vi "CTRE_Phoenix_MotorControl_BufferedTrajectoryPointStream_Clear.vi"(8 "error in":errorcluster, 11 "BufferedTrajectoryPointStream_DevRef":T1) -> (0 "error out":errorcluster, 3 "BufferedTrajectoryPointStream_DevRef":T1)   [LabVIEW 2020]
doc: "Clears the Buffered Trajectory Point Stream"
uses:
  <vilib>/Rock Robotics/WPI/ThirdParty/Phoenix-LabVIEW/Motor Controller/Controls/CTRE_Phoenix_MotorControl_BufferedTrajectoryPointStream_DeviceRef.ctl
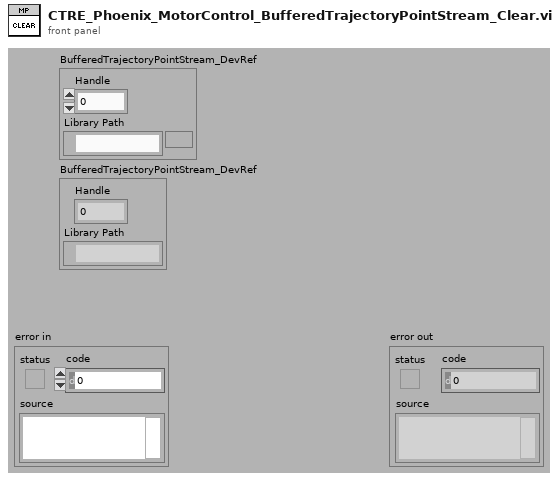
[diagram p1: front panel]
types:
  T1 = typedef "CTRE_Phoenix_MotorControl_BufferedTrajectoryPointStream_DeviceRef.ctl" = cluster{"Handle":u64, "Library Path":path}
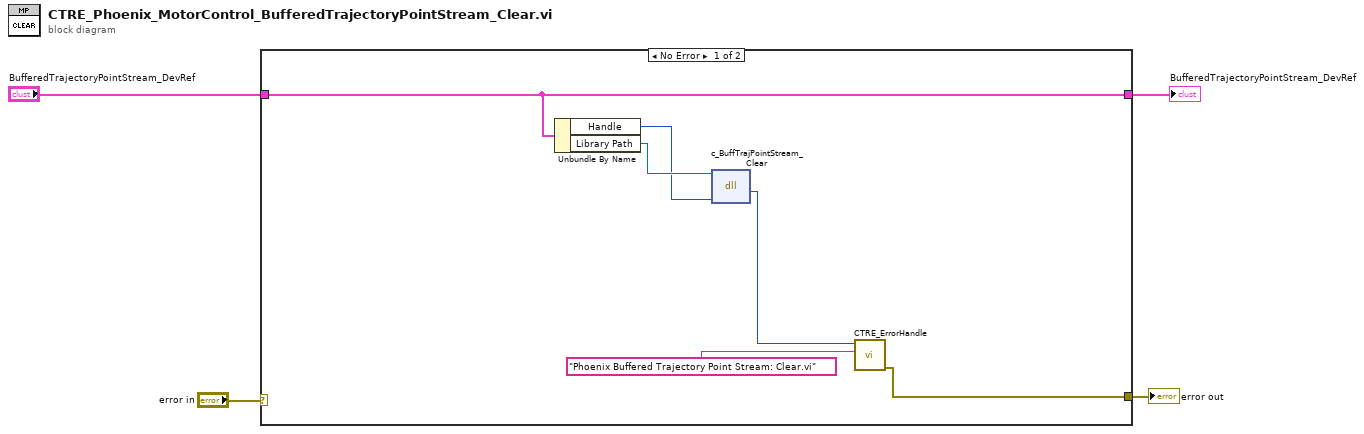
[diagram p0: block diagram]
diagram:
  n1 = case shown="No Error" "error in" {
    selector: "error in" -> [_ w12]
    tunnel: [w5 w12] -> w4
    tunnel: [w10 w11] -> w1
    tunnel: "BufferedTrajectoryPointStream_DevRef" -> [w10 w11]
    frame No Error {
      n2 = Unbundle By Name(w10) -> ("Handle"=w8:u64, "Library Path"=w9:path)
      n3 = dll-call lib="?" fn="c_BuffTrajPointStream_Clear"(path in=w9, "handle"=w8) -> ("ErrorCode"=w6:i32)  [unwired: 3 in, 2 out]
      n4 = call <vilib>:"CTRE_ErrorHandle.vi"("origin"="Phoenix Buffered Trajectory Point Stream: Clear.vi", "code"=w6) -> ("error out"=w5:errorcluster)  [unwired: 9 in]
    }
    frame Error {
    }
  }
  "error out" <- w4
  "BufferedTrajectoryPointStream_DevRef" <- w1
